vi "fgm_pipeline_partial.vi"(6 "du_max":fxp<+/-,18,1>, 8 "x_vec":T3=[0.0, 0.0, 0.0, 0.0, 0.0, 0.0, 0.0, 0.0, 0.0, 0.0, 0.0, 0.0, 0.0, 0.0, 0.0, 0.0, 0.0, 0.0, 0.0, 0.0, 0.0, 0.0, 0.0, 0.0, 0.0], 11 "QP_params":T4={"maxIter"=0, "nuN"=24, "Ns_mpc"=0, "-beta"=-0.9987945556640625, "beta+1"=1.9987945556640625}) -> (1 "delta u(k)":fxp<+/-,32,3>)   [LabVIEW 2017]
uses:
  quadProgParams_pipe.ctl
  x_vec_type_pipe.ctl
  x_qp_scalar.ctl
  ziyi_pipe.ctl
  xtype_scalar.ctl
  <vilib>/rvi/Emulation/niFpgaEmulationIsFPGAContextNoSignature.vi
  <vilib>/rvi/DataTransferAndStorage/Container/Common/niFpgaContainerGetUniqueNameForEmu.vi
  <vilib>/rvi/Memory/Memory_Emulation/niFpgaMemoryEmulationCacheClearOnFirstRun.vi
  <vilib>/rvi/Memory/Memory_Emulation/nirvimemoryEmulationManagerCache_MakeExclusive.vi
  <vilib>/rvi/Memory/Memory_Emulation/niFpgaMemoryEmulationValidateCache.vi
  <vilib>/rvi/Memory/Memory_Emulation/nirvimemoryEmulationManagerCache_InsertValue.vi
  <vilib>/Utility/error.llb/Clear Errors.vi
  <vilib>/rvi/Memory/Memory_Emulation/nirvimemoryEmulationManagerCache_ReleaseExclusive.vi
  <vilib>/rvi/Memory/Memory_Emulation/nirvimemoryEmulationManagerCache_GetValue.vi
  <vilib>/rvi/Memory/Memory_Emulation/nirvimemoryEmulationManagerCache_SetValue.vi
  <vilib>/rvi/Emulation/niFpgaProcessEmulError.vi
  <vilib>/rvi/Emulation/niFpgaSctlEmulationGetInTimedLoop.vi
  <vilib>/rvi/DataTransferAndStorage/Container/XNode/niFpgaContainer.xnode
  <vilib>/rvi/DataTransferAndStorage/Register/Emulation/niFpgaRegisterEmulation.vi
panel:
  out "z":T1
  out "y":T1
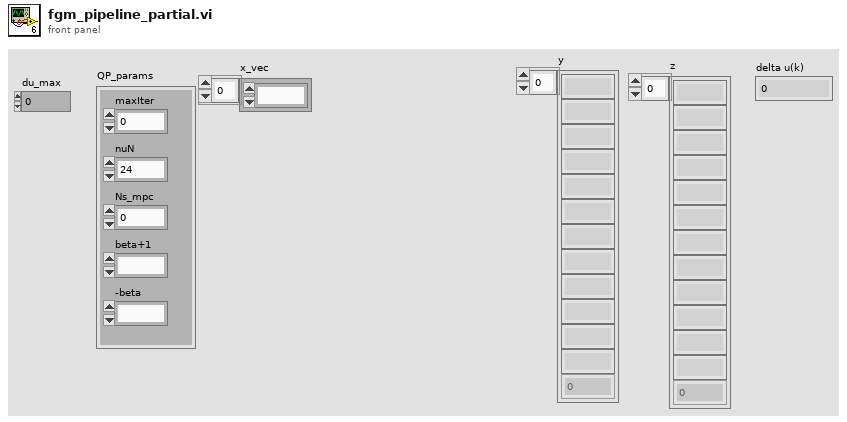
[diagram p1: front panel]
types:
  T1 = typedef "ziyi_pipe.ctl" = T2[]
  T2 = typedef "x_qp_scalar.ctl" = fxp<+/-,32,6>
  T3 = typedef "x_vec_type_pipe.ctl" = T2[]
  T4 = typedef "quadProgParams_pipe.ctl" = cluster{"maxIter":u16, "nuN":u16, "Ns_mpc":u16, "-beta":fxp<+/-,18,2>, "beta+1":fxp<+/-,18,2>}
  T5 = typedef "xtype_scalar.ctl" = fxp<+/-,32,6>
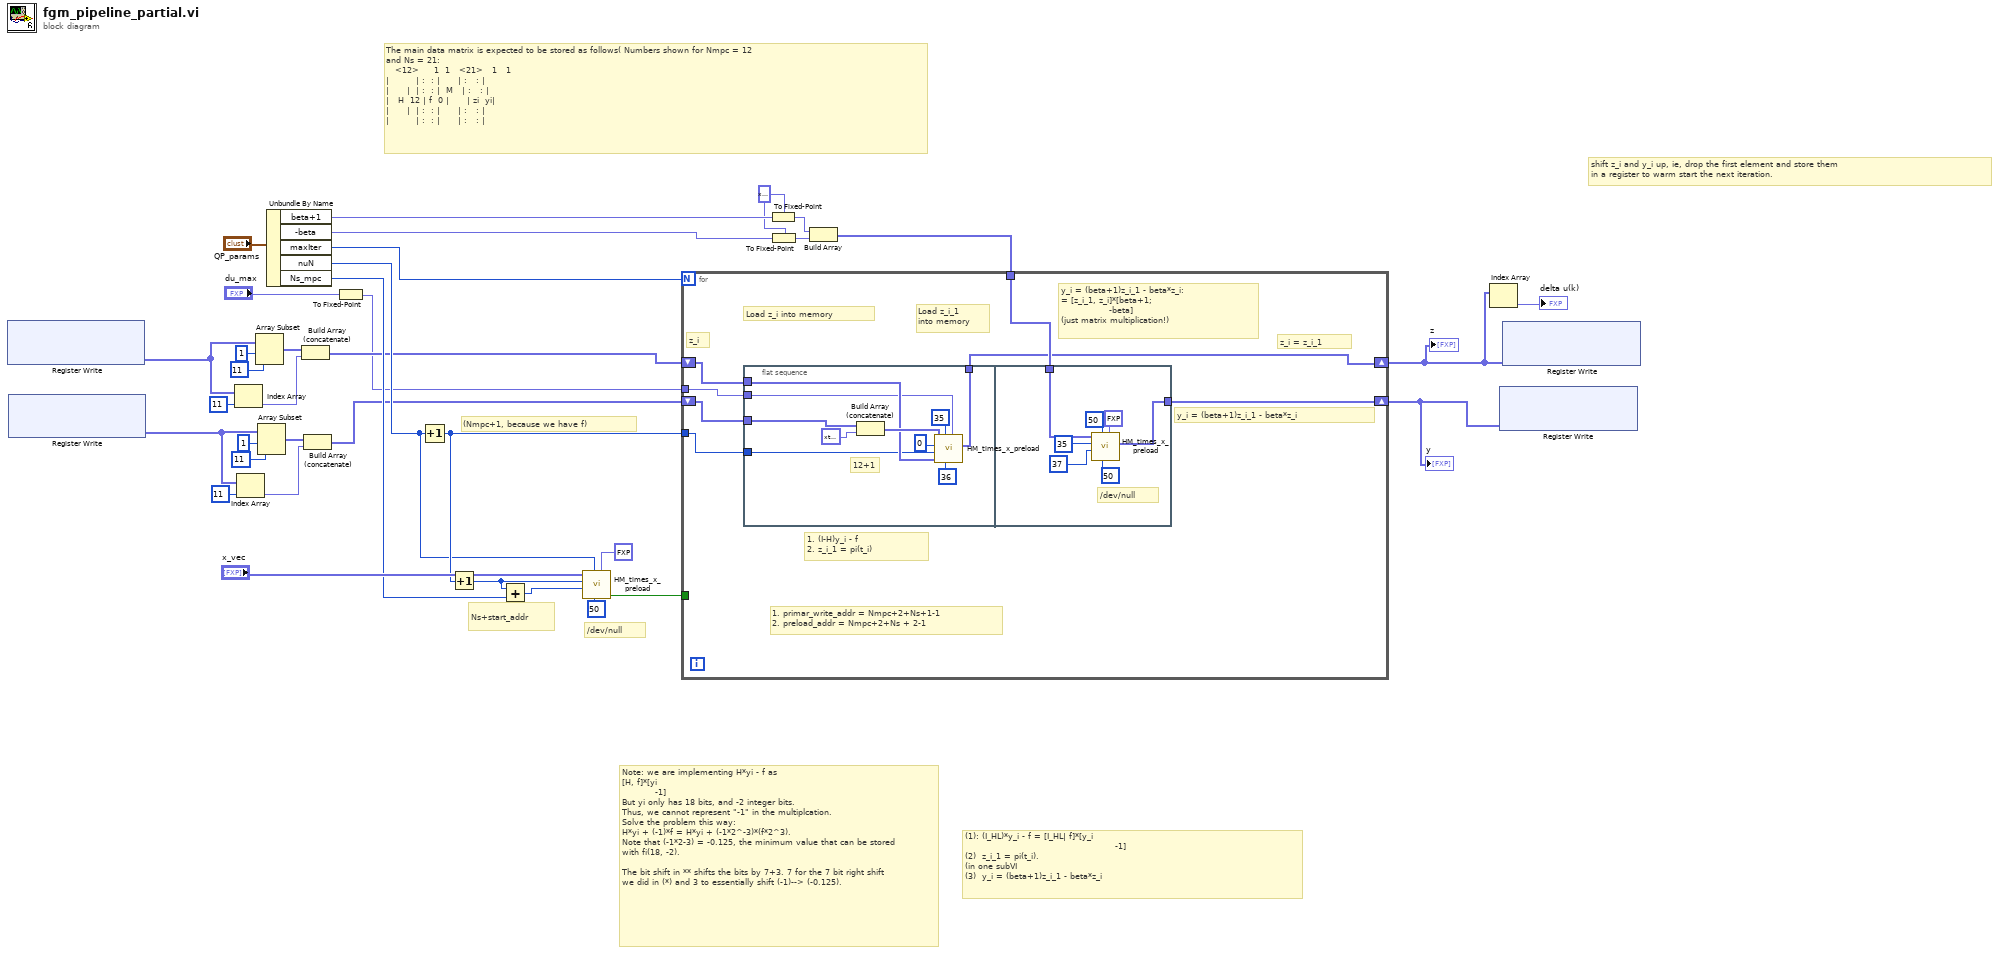
[diagram p0: block diagram]
diagram:
  w7 = T5 0.0 ("xtype")
  # "The main data matrix is expected to be stored as follows( Numbers shown for Nmpc = 12\nand Ns = 21:\n   <12>     1  1   <21>   1   1\n|         | :  : |      | :   : |\n|      |  | :  : |  M   | :   : |\n|   H  12 | f  0 |      | zi  yi|\n|      |  | :  : |      | :   : |\n|         | :  : |      | :   : |"
  # "Ns+start_addr"
  # "(Nmpc+1, because we have f)"
  # "/dev/null"
  # "Note: we are implementing H*yi - f as\n[H, f]*[yi\n           -1]\nBut yi only has 18 bits, and -2 integer bits. \nThus, we cannot represent \"-1\" in the multiplcation.\nSolve the problem this way:\nH*yi + (-1)*f = H*yi + (-1*2^-3)*(f*2^3).\nNote that (-1*2-3) = -0.125, the minimum value that can be stored\nwith fi(18, -2).\n\nThe bit shift in ** shifts the bits by 7+3. 7 for the 7 bit right shift\nwe did in (*) and 3 to essentially shift (-1)--> (-0.125)."
  # "(1): (I_HL)*y_i - f = [I_HL| f]*[y_i\n                                                  -1]\n(2)  z_i_1 = pi(t_i).\n(in one subVI\n(3)  y_i = (beta+1)z_i_1 - beta*z_i"
  # "shift z_i and y_i up, ie, drop the first element and store them\nin a register to warm start the next iteration."
  n1 = xnode "Register Write"() -> ("Data"=w4:fxp<+/-,32,6>[])  [unwired: 1 in, 1 out]
  n2 = xnode "Register Write"() -> ("Data"=w3:fxp<+/-,32,6>[])  [unwired: 1 in, 1 out]
  n3 = Index Array(array=w4, index=11) -> (element=w10:fxp<+/-,32,6>)
  n4 = Index Array(array=w3, index=11) -> (element=w11:fxp<+/-,32,6>)
  n5 = Array Subset(array=w4, index=1, length=11) -> (w16:fxp<+/-,32,6>[])
  n6 = Array Subset(array=w3, index=1, length=11) -> (w12:fxp<+/-,32,6>[])
  n7 = Unbundle By Name("QP_params") -> ("beta+1"=w34:fxp<+/-,18,2>, "-beta"=w33:fxp<+/-,18,2>, "maxIter"=w35:u16, "nuN"=w22:u16, "Ns_mpc"=w21:u16)
  n8 = Build Array (concatenate)(w16, w10) -> (w9:fxp<+/-,32,6>[])
  n9 = Build Array (concatenate)(w12, w11) -> (w8:fxp<+/-,32,6>[])
  n10 = To Fixed-Point(number="du_max") -> (fixed-point=w6:fxp<+/-,18,5>)  [unwired: 1 in]
  n11 = Increment(x=w22) -> (x+1=w26:u16)
  n12 = Increment(x=w26) -> (x+1=w24:u16)
  n13 = Add(x=w24, y=w21) -> (x+y=w23:u16)
  n14 = call "HM_times_x_preload.vi"("SLMAX"=fxp<+/-,18,5> 15.9998779296875, "preload_addr"=u8 50, "primary_write_addr"=w22, "Ns+StartIndex"=w23, "StartIndex"=w24, "x_vec"="x_vec") -> ("done"=w29:bool)  [unwired: 4 in, 1 out]
  n15 = To Fixed-Point(fixed-point type=w7, number=w34) -> (fixed-point=w31:T5)
  n16 = To Fixed-Point(fixed-point type=w7, number=w33) -> (fixed-point=w30:T5)
  n17 = Build Array(w31, w30) -> (w27:T5[])
  n18 = for {
    N: w35 -> [_]
    shift-right: [w42] -> w2
    shift-left: w8 -> [w41]
    shift-right: [w38] -> w1
    shift-left: w9 -> [w37]
    tunnel: w27 -> [w43]
    tunnel: w6 -> [w39]
    tunnel: w29 -> [_]
    tunnel: w26 -> [w40]
    # "1. primar_write_addr = Nmpc+2+Ns+1-1\n2. preload_addr = Nmpc+2+Ns + 2-1"
    # "y_i = (beta+1)z_i_1 - beta*z_i:\n= [z_i_1, z_i]*[beta+1;\n                -beta]\n(just matrix multiplication!)"
    # "Load z_i into memory"
    # "Load z_i_1\ninto memory"
    # "1. (I-H)y_i - f\n2. z_i_1 = pi(t_i)"
    # "z_i = z_i_1"
    # "y_i = (beta+1)z_i_1 - beta*z_i"
    # "z_i"
    n19 = flat-sequence {
      tunnel: w37 -> [w49]
      tunnel: w41 -> [w48]
      tunnel: w40 -> [w47]
      tunnel: w39 -> [w46]
      tunnel: [w45] -> w38
      tunnel: w43 -> [w60]
      tunnel: [w56] -> w42
      frame #0 {
        # "12+1"
        n20 = Build Array (concatenate)(w48, T5 -1.0 ("xtype")) -> (w50:T5[])
        n21 = call "HM_times_x_preload.vi"("SLMAX"=w46, "preload_addr"=u8 36 ("Address (Max = 255)"), "primary_write_addr"=u8 35 ("Address (Max = 255)"), "preload_vec"=w49, "Ns+StartIndex"=w47, "StartIndex"=u8 0 ("rowOffset"), "x_vec"=w50) -> ("A*x"=w45:T1)  [unwired: 3 in, 1 out]
      }
      frame #1 {
        # "/dev/null"
        n22 = call "HM_times_x_preload.vi"("SLMAX"=fxp<+/-,18,5> 15.9998779296875, "preload_addr"=u8 50, "primary_write_addr"=u8 50, "Ns+StartIndex"=u16 37 ("Ncols"), "StartIndex"=u8 35 ("MatrixStartIndex"), "x_vec"=w60) -> ("A*x"=w56:T1)  [unwired: 4 in, 1 out]
      }
    }
  }
  "y" <- w2
  "z" <- w1
  n23 = Index Array(array=w1) -> (element=→"delta u(k)":T2)  [unwired: 1 in]
  n24 = xnode "Register Write"("Data"=w2) -> ()  [unwired: 1 in, 1 out]
  n25 = xnode "Register Write"("Data"=w1) -> ()  [unwired: 1 in, 1 out]
